vi "Max HovaCAL MFCs Pumps.vi"() -> (2 "max Pumps":i32, 3 "max MFCs":i32)   [LabVIEW 2020, in "Linearisierung v2.lvlib" / "Gasteiler.lvlib" / "HovaCAL_Interface.lvlib" / "Kommunikation.lvlib"]
uses:
  Kommunikation/Kommunikation.lvlib
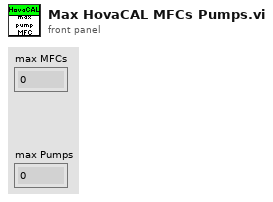
[diagram p1: front panel]
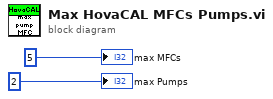
[diagram p0: block diagram]
diagram:
  "max MFCs" <- 5 ("Index")
  "max Pumps" <- 2 ("Länge")
